vi "GetFilterFromTreeVal.vi"(10 "Value":string, 11 "Tree Ref In":refnum<vi>) -> (2 "Filter":string, 3 "Tree Ref Out":refnum<vi>)   [LabVIEW 2016, in "NI_NPW_Filters.lvlib"]
uses:
  <resource>/dialog/NewProjectWizard/Filters/NI_NPW_Filters.lvlib
panel:
  in  "Test Tree":string(tree)
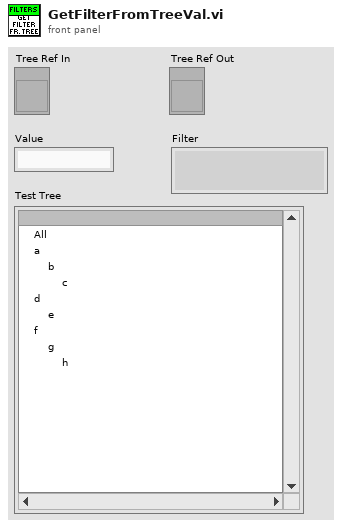
[diagram p1: front panel]
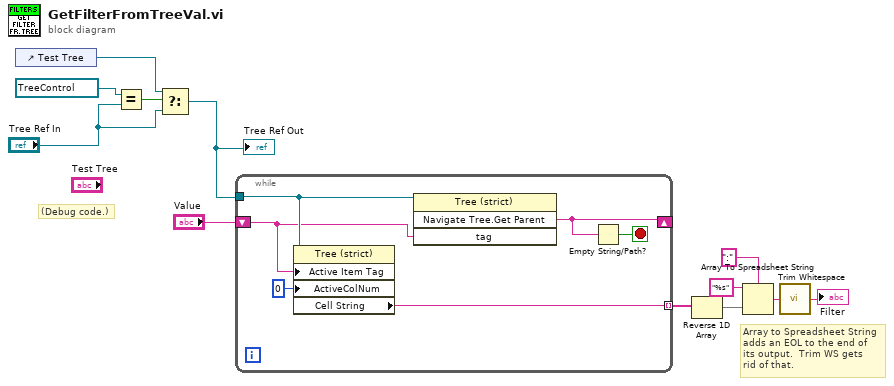
[diagram p0: block diagram]
diagram:
  # "Array to Spreadsheet String\nadds an EOL to the end of\nits output.  Trim WS gets\nrid of that."
  # "(Debug code.)"
  n1 = control-ref of="Test Tree"() -> (w6:refnum<vi>)
  n2 = Equal?(x=refnum<vi> refnum ("Tree Refnum"), y="Tree Ref In") -> (x = y?=w8:bool)
  n3 = Select(t=w6, s=w8, f="Tree Ref In") -> (s? t:f=w4:refnum<vi>)
  "Tree Ref Out" <- w4
  n4 = while {
    tunnel: w4 -> [w17]
    tunnel: [w18] -> w2 mode=indexing
    shift-right: [w14] -> _
    shift-left: "Value" -> [w16]
    stop <- w15 stop-if-true
    n5 = property class="Tree (strict)"(reference=w17, "Active Item Tag"=w16, "ActiveColNum"=0 ("Active Cell:Active Column Number")) -> ("Cell String"=w18:string)  [unwired: 1 in, 2 out]
    n6 = invoke class="Tree (strict)" method="Navigate Tree.Get Parent"(reference=w17, "tag"=w16) -> ("Navigate Tree:Get Parent"=w14:string)  [unwired: 2 in, 3 out]
    n7 = Empty String/Path?(string/path=w14) -> (empty?=w15:bool)
  }
  n8 = Reverse 1D Array(array=w2) -> (reversed array=w11:string[])
  n9 = Array To Spreadsheet String(delimiter (Tab)=":", array=w11, 3:"%s" ("format string")) -> (spreadsheet string=w3:string)
  n10 = call <vilib>:"Trim Whitespace.vi"("string"=w3) -> ("trimmed string"=→"Filter":string)  [unwired: 1 in]
